vi "arreglos.vi"(0 "Orden":T2(array[ring])=[enum."espejos", enum."voltaje", enum."polarizador", enum."potenciometro ", enum."CCD"], 1 "DISP 1":i32, 2 "Cluster DISP 1":T1, 3 "DISP 2":i32, 4 "DISP 3":i32, 5 "DISPLONG 1":i32, 6 "Cluster DISP 2":T1, 7 "DISPLONG 2":i32, 8 "DISPLONG 3":i32, 9 "nombre":string, 10 "CORRIENTE":dbl[](array[numeric]), 11 "MULTIMETRO 2":dbl[](array[numeric]), 12 "VOLTAJE":dbl[](array[numeric]), 13 "X":dbl[](array[numeric]), 14 "ANGULO":dbl[](array[numeric]), 15 "Y":dbl[](array[numeric]), 16 "laser":dbl[](array[numeric]), 17 "POTENCIOMETRO":dbl[](array[numeric]), 18 "LOCKIN":dbl[](array[numeric]), 19 "CCD":dbl[][](array[numeric]), 20 "MULTIMETRO":bool, 24 "Cluster DISP 4":T1, 27 "Cluster DISP 3":T1) -> (21 "disp 2":T1, 23 "disp 1":T1, 25 "disp 3":T1, 26 "disp 4":T1)   [LabVIEW 2016]
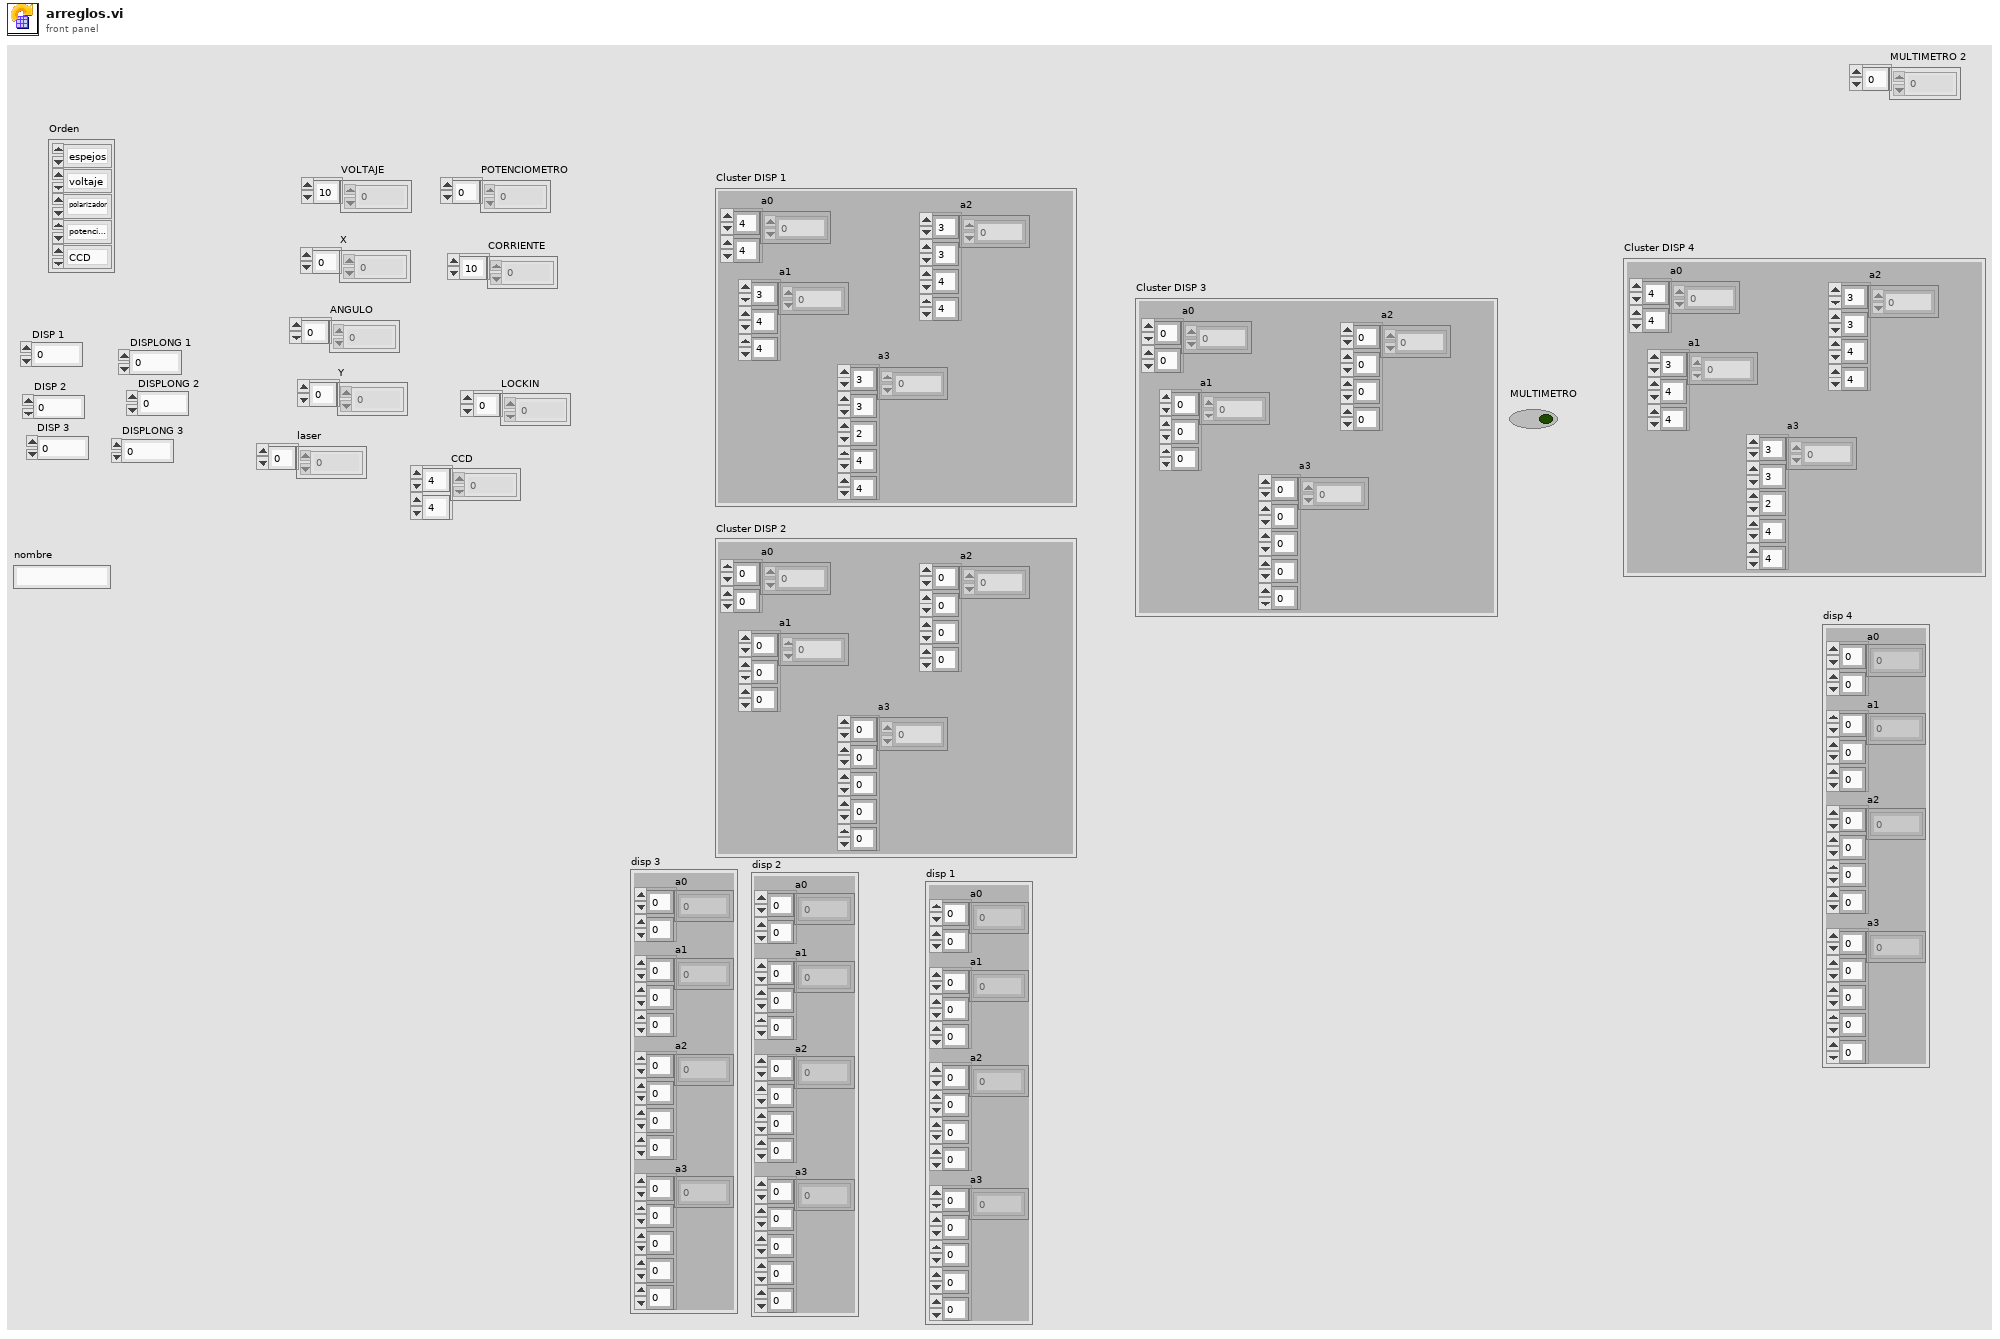
[diagram p1: front panel]
types:
  T1 = cluster{"a0":dbl[][], "a1":dbl[][][], "a2":dbl[][][][], "a3":dbl[][][][][]}
  T2 = enum16{"espejos", "polarizador", "voltaje", "potenciometro ", "CCD", "lockin", "laser", "ninguno"}[]
  T3 = enum16{"espejos", "polarizador", "voltaje", "potenciometro ", "CCD", "lockin", "laser", "ninguno"}
  T4 = enum16{"espejos", "polarizador", "voltaje", "potenciometro ", "CCD", "lockin", "laser", "multimetro", "ninguno"}
  T5 = cluster{"a0":dbl[][], "a1":dbl[][][], "a2":dbl[][][][], "a3":dbl[][][][][]}[]
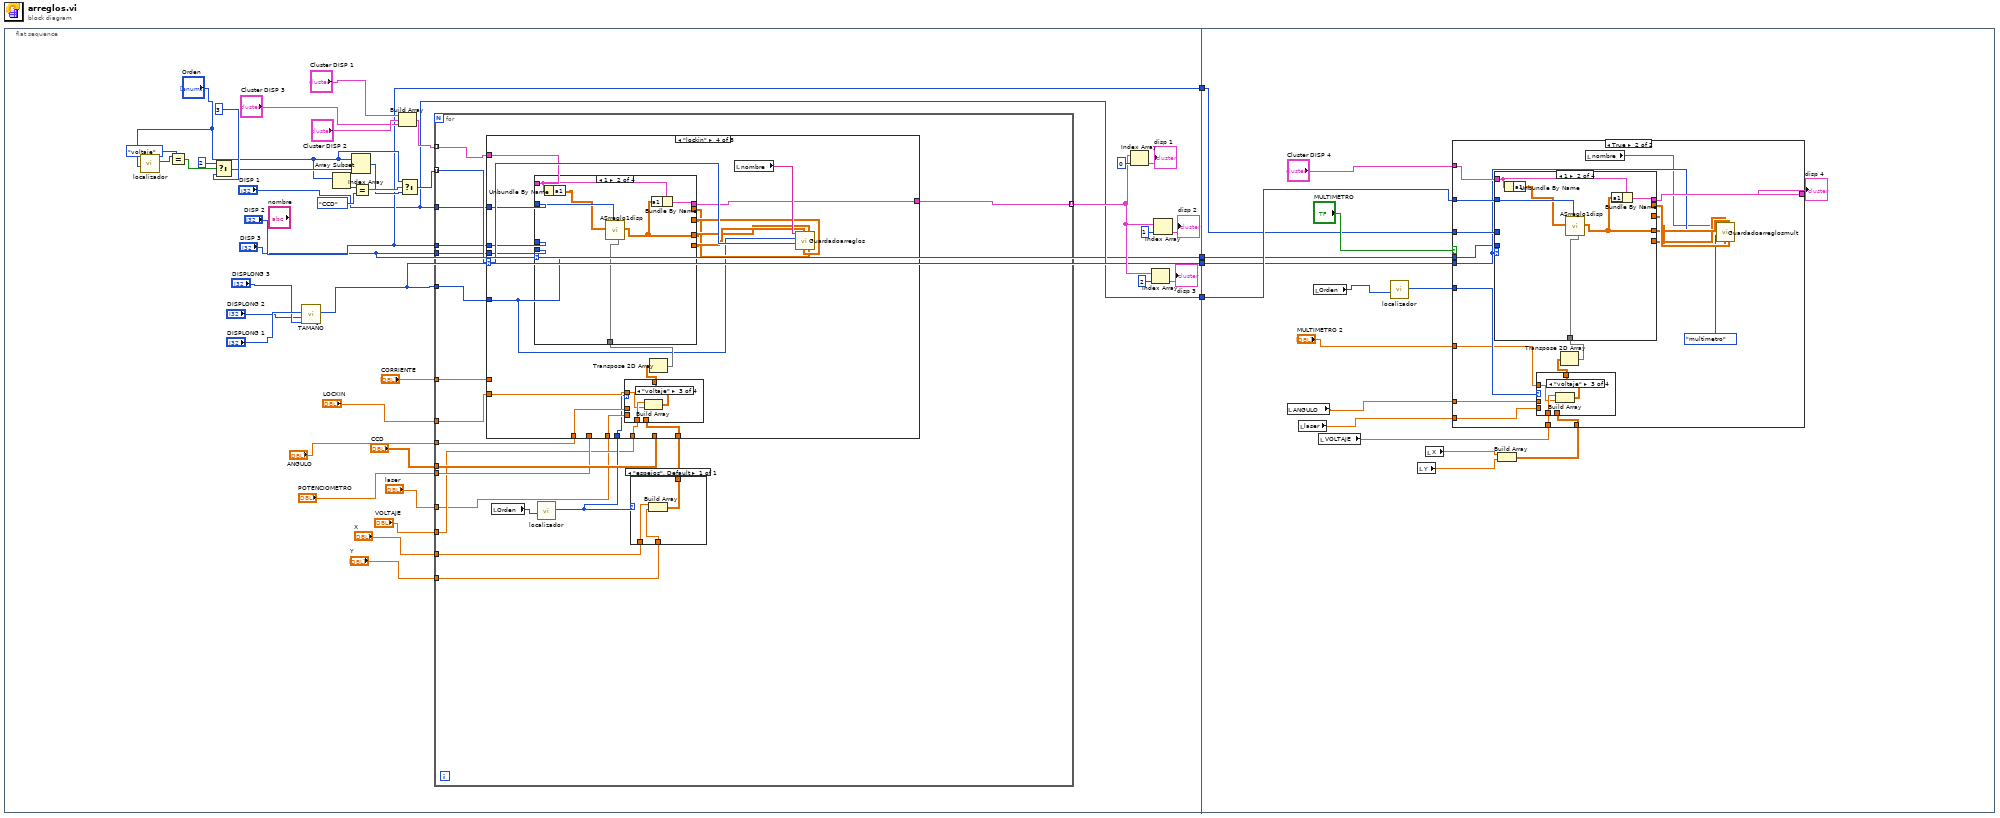
[diagram p0: block diagram]
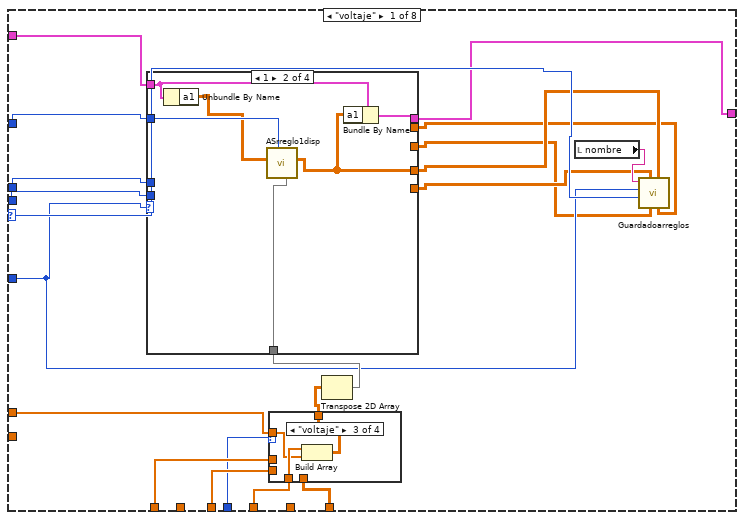
[diagram p2: hidden frame]
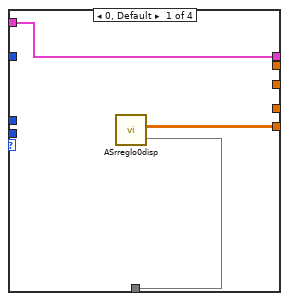
[diagram p3: hidden frame]
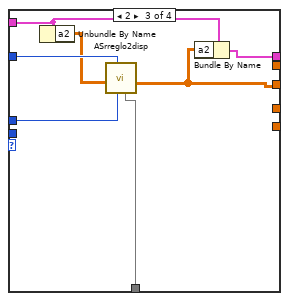
[diagram p4: hidden frame]
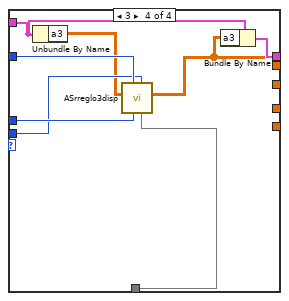
[diagram p5: hidden frame]
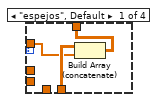
[diagram p6: hidden frame]
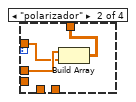
[diagram p7: hidden frame]
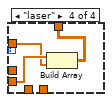
[diagram p8: hidden frame]
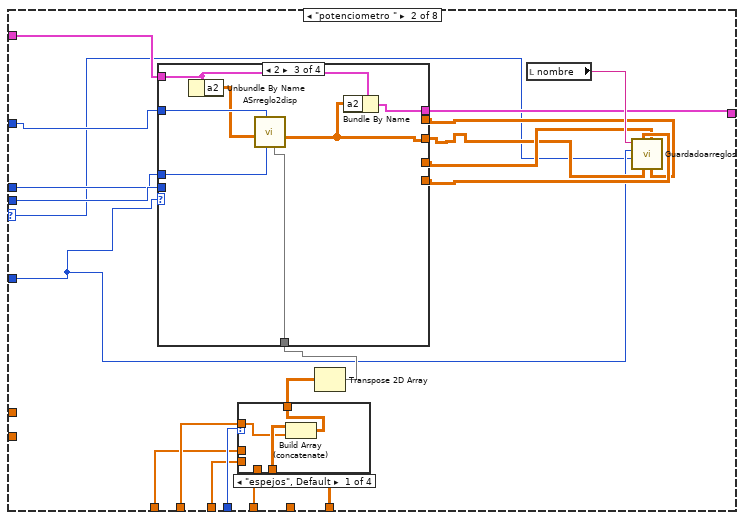
[diagram p9: hidden frame]
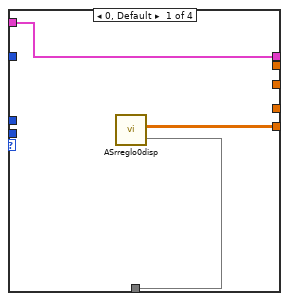
[diagram p10: hidden frame]
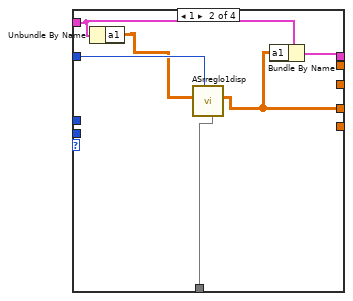
[diagram p11: hidden frame]
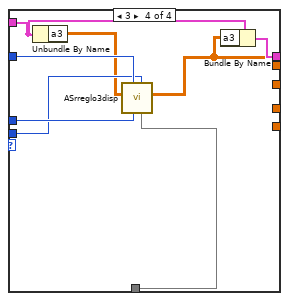
[diagram p12: hidden frame]
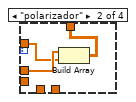
[diagram p13: hidden frame]
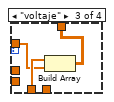
[diagram p14: hidden frame]
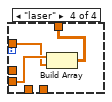
[diagram p15: hidden frame]
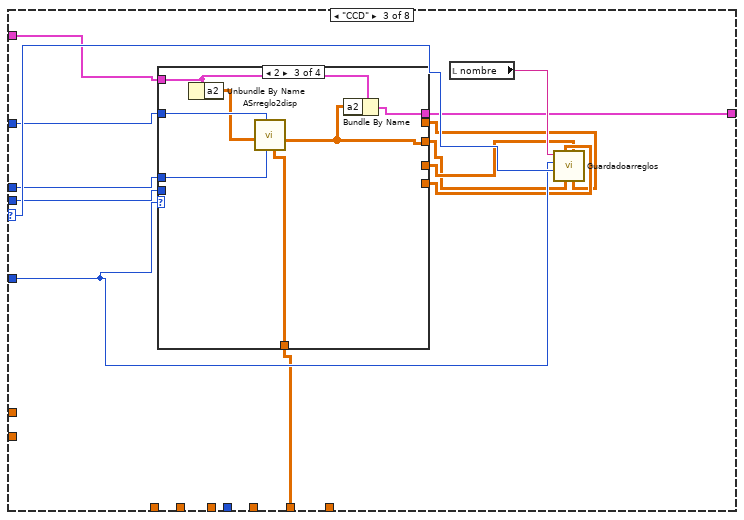
[diagram p16: hidden frame]
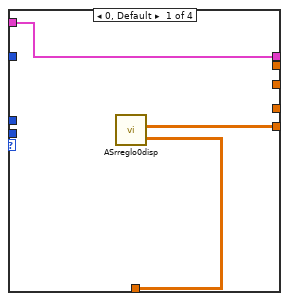
[diagram p17: hidden frame]
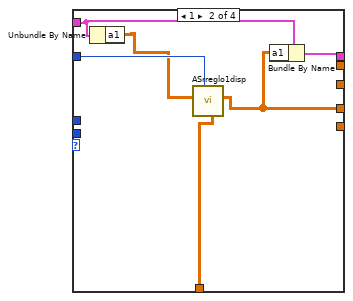
[diagram p18: hidden frame]
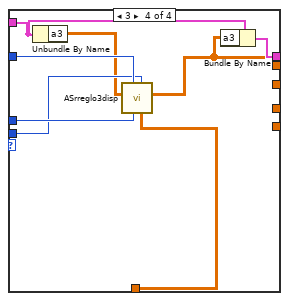
[diagram p19: hidden frame]
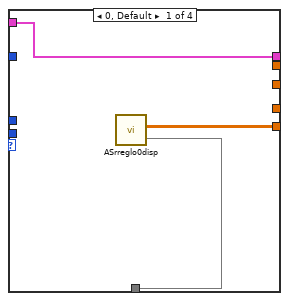
[diagram p20: hidden frame]
diagram:
  n1 = flat-sequence {
    tunnel: ["DISP 1"] -> w4
    tunnel: ["DISP 2"] -> w3
    tunnel: [w7] -> w2
    tunnel: ["DISP 3"] -> w1
    tunnel: w4 -> [w278]
    tunnel: w3 -> [w277]
    tunnel: w2 -> [w276]
    tunnel: w1 -> [w275]
    frame #0 {
      n2 = call "localizador.vi"("Orden"="Orden") -> ("Enum"=w24:T3)  [unwired: 9 in, 1 out]
      n3 = Equal?(x=w24, y=T3."voltaje") -> (x = y?=w22:bool)
      n4 = Select(t=2, s=w22, f=3 ("index")) -> (s? t:f=w20:i32)
      n5 = call "TAMAÑO.vi"("DISPLONG 3"="DISPLONG 3", "DISPLONG 2"="DISPLONG 2", "DISPLONG 1"="DISPLONG 1") -> ("result"=w7:i32)  [unwired: 8 in]
      n6 = Index Array(array="Orden") -> (element=w14:T3)  [unwired: 1 in]
      n7 = Array Subset(array="Orden", index=w20) -> (w10:T2)  [unwired: 1 in]
      n8 = Equal?(x=w14, y=T3."CCD") -> (x = y?=w12:bool)
      n9 = Build Array("Cluster DISP 1", "Cluster DISP 2", "Cluster DISP 3") -> (w29:T5)
      n10 = Select(t="Orden", s=w12, f=w10) -> (s? t:f=w9:T2)
      n11 = for {
        tunnel: w9 -> [w61] mode=indexing
        tunnel: w7 -> [w62]
        tunnel: "CCD" -> [w60]
        tunnel: "DISP 1" -> [w59]
        tunnel: "DISP 2" -> [w58]
        tunnel: "DISP 3" -> [w57]
        tunnel: "POTENCIOMETRO" -> [w56]
        tunnel: "Y" -> [w54]
        tunnel: "X" -> [w53]
        tunnel: "VOLTAJE" -> [w50]
        tunnel: "ANGULO" -> [w49]
        tunnel: "laser" -> [w48]
        tunnel: "LOCKIN" -> [w47]
        tunnel: "CORRIENTE" -> [w46]
        tunnel: w29 -> [w45] mode=indexing
        tunnel: [w44] -> w17 mode=indexing
        n12 = local read "Orden"() -> (w55:T2)
        n13 = call "localizador.vi"("Orden"=w55) -> ("Enum"=w51:T3)  [unwired: 9 in, 1 out]
        n14 = case shown="\"espejos\", Default" w51 {
          tunnel: w54 -> [w64]
          tunnel: w53 -> [w65]
          tunnel: [w63] -> w52
          frame "espejos", Default {
            n15 = Build Array(w65, w64) -> (w63:dbl[][])
          }
        }
        n16 = case shown="\"lockin\"" w61 {
          selector: w61 -> [w77 w122 w189 w226 _ _ _ _]
          tunnel: w62 -> [w75 w126 w185 w215 _ _ _ _]
          tunnel: w60 -> [_ _ w184 _ _ _ _ _]
          tunnel: w59 -> [w72 w123 w188 w223 _ _ _ _]
          tunnel: w58 -> [w73 w124 w187 w225 _ _ _ _]
          tunnel: w57 -> [w74 w125 w186 w224 _ _ _ _]
          tunnel: w56 -> [_ w141 _ _ _ _ _ _]
          tunnel: w52 -> [w80 w140 _ w231 _ _ _ _]
          tunnel: w51 -> [w79 w139 _ w228 _ _ _ _]
          tunnel: w50 -> [w82 w138 _ w229 _ _ _ _]
          tunnel: w49 -> [w84 w136 _ w234 _ _ _ _]
          tunnel: w48 -> [w81 w135 _ w230 _ _ _ _]
          tunnel: w47 -> [_ _ _ w233 _ _ _ _]
          tunnel: w46 -> [w83 _ _ _ _ _ _ _]
          tunnel: w45 -> [w71 w129 w179 w222 w271 w272 w273 w274]
          tunnel: [w70 w128 w178 w221 w271 w272 w273 w274] -> w44
          frame "voltaje" {
            n17 = case shown="\"voltaje\"" w79 {
              tunnel: [w110 w113 w116 w119] -> w85
              tunnel: w83 -> [w111 w114 w117 w120]
              tunnel: w80 -> [w112 _ _ _]
              tunnel: w82 -> [_ _ w118 _]
              tunnel: w84 -> [_ w115 _ _]
              tunnel: w81 -> [_ _ _ w121]
              frame "espejos", Default {
                n18 = Build Array (concatenate)(w112, w111) -> (w110:dbl[][])
              }
              frame "polarizador" {
                n19 = Build Array(w115, w114) -> (w113:dbl[][])
              }
              frame "voltaje" {
                n20 = Build Array(w118, w117) -> (w116:dbl[][])
              }
              frame "laser" {
                n21 = Build Array(w121, w120) -> (w119:dbl[][])
              }
            }
            n22 = Transpose 2D Array(2D array=w85) -> (transposed array=w76:dbl[][])
            n23 = case shown="1" w75 {
              tunnel: [w88 _ _ _] -> w69
              tunnel: w76 -> [w87 w93 w101 w109]
              tunnel: [_ w89 _ _] -> w68
              tunnel: [_ _ w97 _] -> w67
              tunnel: [_ _ _ w102] -> w66
              tunnel: w72 -> [_ w94 w100 w107]
              tunnel: w73 -> [_ _ w95 w108]
              tunnel: w74 -> [_ _ _ w106]
              tunnel: w71 -> [w86 w90 w98 w103]
              tunnel: [w86 w91 w96 w104] -> w70
              frame 0, Default {
                n24 = call "ASrreglo0disp.vi"("datos"=w87) -> ("output array"=w88:dbl[][])  [unwired: 10 in]
              }
              frame 1 {
                n25 = Unbundle By Name(w90) -> ("a1"=w92:dbl[][][])
                n26 = call "ASrreglo1disp.vi"("datos"=w93, "disp. 1"=w94, "ARREGLO ENTRADA"=w92) -> ("output array"=w89:dbl[][][])  [unwired: 8 in]
                n27 = Bundle By Name(cluster=w90, "a1"=w89) -> (w91:T1)
              }
              frame 2 {
                n28 = Unbundle By Name(w98) -> ("a2"=w99:dbl[][][][])
                n29 = call "ASrreglo2disp.vi"("datos"=w101, "disp. 2"=w95, "disp. 1"=w100, "arreglo entrada"=w99) -> ("output array"=w97:dbl[][][][])  [unwired: 7 in]
                n30 = Bundle By Name(cluster=w98, "a2"=w97) -> (w96:T1)
              }
              frame 3 {
                n31 = Unbundle By Name(w103) -> ("a3"=w105:dbl[][][][][])
                n32 = call "ASrreglo3disp.vi"("datos"=w109, "disp. 3"=w106, "disp. 2"=w108, "disp. 1"=w107, "output array 2"=w105) -> ("output array"=w102:dbl[][][][][])  [unwired: 6 in]
                n33 = Bundle By Name(cluster=w103, "a3"=w102) -> (w104:T1)
              }
            }
            n34 = local read "nombre"() -> (w78:string)
            n35 = call "Guardadoarreglos.vi"("disp 3"=w66, "disp 1"=w68, "disp 2"=w67, "disp 0"=w69, "Enum"=w77, "indice"=w75, "nombre"=w78) -> ()  [unwired: 5 in]
          }
          frame "potenciometro " {
            n36 = case shown="\"espejos\", Default" w139 {
              tunnel: [w166 w169 w172 w175] -> w137
              tunnel: w141 -> [w167 w170 w173 w176]
              tunnel: w140 -> [w168 _ _ _]
              tunnel: w138 -> [_ _ w174 _]
              tunnel: w136 -> [_ w171 _ _]
              tunnel: w135 -> [_ _ _ w177]
              frame "espejos", Default {
                n37 = Build Array (concatenate)(w168, w167) -> (w166:dbl[][])
              }
              frame "polarizador" {
                n38 = Build Array(w171, w170) -> (w169:dbl[][])
              }
              frame "voltaje" {
                n39 = Build Array(w174, w173) -> (w172:dbl[][])
              }
              frame "laser" {
                n40 = Build Array(w177, w176) -> (w175:dbl[][])
              }
            }
            n41 = Transpose 2D Array(2D array=w137) -> (transposed array=w127:dbl[][])
            n42 = case shown="2" w126 {
              tunnel: [w144 _ _ _] -> w133
              tunnel: w127 -> [w143 w149 w157 w165]
              tunnel: [_ w145 _ _] -> w132
              tunnel: [_ _ w153 _] -> w131
              tunnel: [_ _ _ w158] -> w130
              tunnel: w123 -> [_ w150 w156 w163]
              tunnel: w124 -> [_ _ w151 w164]
              tunnel: w125 -> [_ _ _ w162]
              tunnel: w129 -> [w142 w146 w154 w159]
              tunnel: [w142 w147 w152 w160] -> w128
              frame 0, Default {
                n43 = call "ASrreglo0disp.vi"("datos"=w143) -> ("output array"=w144:dbl[][])  [unwired: 10 in]
              }
              frame 1 {
                n44 = Unbundle By Name(w146) -> ("a1"=w148:dbl[][][])
                n45 = call "ASrreglo1disp.vi"("datos"=w149, "disp. 1"=w150, "ARREGLO ENTRADA"=w148) -> ("output array"=w145:dbl[][][])  [unwired: 8 in]
                n46 = Bundle By Name(cluster=w146, "a1"=w145) -> (w147:T1)
              }
              frame 2 {
                n47 = Unbundle By Name(w154) -> ("a2"=w155:dbl[][][][])
                n48 = call "ASrreglo2disp.vi"("datos"=w157, "disp. 2"=w151, "disp. 1"=w156, "arreglo entrada"=w155) -> ("output array"=w153:dbl[][][][])  [unwired: 7 in]
                n49 = Bundle By Name(cluster=w154, "a2"=w153) -> (w152:T1)
              }
              frame 3 {
                n50 = Unbundle By Name(w159) -> ("a3"=w161:dbl[][][][][])
                n51 = call "ASrreglo3disp.vi"("datos"=w165, "disp. 3"=w162, "disp. 2"=w164, "disp. 1"=w163, "output array 2"=w161) -> ("output array"=w158:dbl[][][][][])  [unwired: 6 in]
                n52 = Bundle By Name(cluster=w159, "a3"=w158) -> (w160:T1)
              }
            }
            n53 = local read "nombre"() -> (w134:string)
            n54 = call "Guardadoarreglos.vi"("disp 3"=w130, "disp 1"=w132, "disp 2"=w131, "disp 0"=w133, "Enum"=w122, "indice"=w126, "nombre"=w134) -> ()  [unwired: 5 in]
          }
          frame "CCD" {
            n55 = case shown="2" w185 {
              tunnel: [w193 _ _ _] -> w183
              tunnel: w184 -> [w192 w198 w206 w214]
              tunnel: [_ w194 _ _] -> w182
              tunnel: [_ _ w202 _] -> w181
              tunnel: [_ _ _ w207] -> w180
              tunnel: w188 -> [_ w199 w205 w212]
              tunnel: w187 -> [_ _ w200 w213]
              tunnel: w186 -> [_ _ _ w211]
              tunnel: w179 -> [w191 w195 w203 w208]
              tunnel: [w191 w196 w201 w209] -> w178
              frame 0, Default {
                n56 = call "ASrreglo0disp.vi"("datos"=w192) -> ("output array"=w193:dbl[][])  [unwired: 10 in]
              }
              frame 1 {
                n57 = Unbundle By Name(w195) -> ("a1"=w197:dbl[][][])
                n58 = call "ASrreglo1disp.vi"("datos"=w198, "disp. 1"=w199, "ARREGLO ENTRADA"=w197) -> ("output array"=w194:dbl[][][])  [unwired: 8 in]
                n59 = Bundle By Name(cluster=w195, "a1"=w194) -> (w196:T1)
              }
              frame 2 {
                n60 = Unbundle By Name(w203) -> ("a2"=w204:dbl[][][][])
                n61 = call "ASrreglo2disp.vi"("datos"=w206, "disp. 2"=w200, "disp. 1"=w205, "arreglo entrada"=w204) -> ("output array"=w202:dbl[][][][])  [unwired: 7 in]
                n62 = Bundle By Name(cluster=w203, "a2"=w202) -> (w201:T1)
              }
              frame 3 {
                n63 = Unbundle By Name(w208) -> ("a3"=w210:dbl[][][][][])
                n64 = call "ASrreglo3disp.vi"("datos"=w214, "disp. 3"=w211, "disp. 2"=w213, "disp. 1"=w212, "output array 2"=w210) -> ("output array"=w207:dbl[][][][][])  [unwired: 6 in]
                n65 = Bundle By Name(cluster=w208, "a3"=w207) -> (w209:T1)
              }
            }
            n66 = local read "nombre"() -> (w190:string)
            n67 = call "Guardadoarreglos.vi"("disp 3"=w180, "disp 1"=w182, "disp 2"=w181, "disp 0"=w183, "Enum"=w189, "indice"=w185, "nombre"=w190) -> ()  [unwired: 5 in]
          }
          frame "lockin" {
            n68 = case shown="\"voltaje\"" w228 {
              tunnel: [w259 w262 w265 w268] -> w232
              tunnel: w233 -> [w260 w263 w266 w269]
              tunnel: w231 -> [w261 _ _ _]
              tunnel: w229 -> [_ _ w267 _]
              tunnel: w234 -> [_ w264 _ _]
              tunnel: w230 -> [_ _ _ w270]
              frame "espejos", Default {
                n69 = Build Array (concatenate)(w261, w260) -> (w259:dbl[][])
              }
              frame "polarizador" {
                n70 = Build Array(w264, w263) -> (w262:dbl[][])
              }
              frame "voltaje" {
                n71 = Build Array(w267, w266) -> (w265:dbl[][])
              }
              frame "laser" {
                n72 = Build Array(w270, w269) -> (w268:dbl[][])
              }
            }
            n73 = Transpose 2D Array(2D array=w232) -> (transposed array=w220:dbl[][])
            n74 = case shown="1" w215 {
              tunnel: [w237 _ _ _] -> w219
              tunnel: w220 -> [w236 w242 w250 w258]
              tunnel: [_ w238 _ _] -> w218
              tunnel: [_ _ w246 _] -> w217
              tunnel: [_ _ _ w251] -> w216
              tunnel: w223 -> [_ w243 w249 w256]
              tunnel: w225 -> [_ _ w244 w257]
              tunnel: w224 -> [_ _ _ w255]
              tunnel: w222 -> [w235 w239 w247 w252]
              tunnel: [w235 w240 w245 w253] -> w221
              frame 0, Default {
                n75 = call "ASrreglo0disp.vi"("datos"=w236) -> ("output array"=w237:dbl[][])  [unwired: 10 in]
              }
              frame 1 {
                n76 = Unbundle By Name(w239) -> ("a1"=w241:dbl[][][])
                n77 = call "ASrreglo1disp.vi"("datos"=w242, "disp. 1"=w243, "ARREGLO ENTRADA"=w241) -> ("output array"=w238:dbl[][][])  [unwired: 8 in]
                n78 = Bundle By Name(cluster=w239, "a1"=w238) -> (w240:T1)
              }
              frame 2 {
                n79 = Unbundle By Name(w247) -> ("a2"=w248:dbl[][][][])
                n80 = call "ASrreglo2disp.vi"("datos"=w250, "disp. 2"=w244, "disp. 1"=w249, "arreglo entrada"=w248) -> ("output array"=w246:dbl[][][][])  [unwired: 7 in]
                n81 = Bundle By Name(cluster=w247, "a2"=w246) -> (w245:T1)
              }
              frame 3 {
                n82 = Unbundle By Name(w252) -> ("a3"=w254:dbl[][][][][])
                n83 = call "ASrreglo3disp.vi"("datos"=w258, "disp. 3"=w255, "disp. 2"=w257, "disp. 1"=w256, "output array 2"=w254) -> ("output array"=w251:dbl[][][][][])  [unwired: 6 in]
                n84 = Bundle By Name(cluster=w252, "a3"=w251) -> (w253:T1)
              }
            }
            n85 = local read "nombre"() -> (w227:string)
            n86 = call "Guardadoarreglos.vi"("disp 3"=w216, "disp 1"=w218, "disp 2"=w217, "disp 0"=w219, "Enum"=w226, "indice"=w215, "nombre"=w227) -> ()  [unwired: 5 in]
          }
          frame "laser" {
          }
          frame "ninguno", Default {
          }
          frame "polarizador" {
          }
          frame "espejos" {
          }
        }
      }
      n87 = Index Array(array=w17, index=0) -> (element=→"disp 1":T1)
      n88 = Index Array(array=w17, index=2) -> (element=→"disp 3":T1)
      n89 = Index Array(array=w17, index=1) -> (element=→"disp 2":T1)
    }
    frame #1 {
      n90 = local read "ANGULO"() -> (w279:dbl[])
      n91 = local read "laser"() -> (w280:dbl[])
      n92 = local read "Orden"() -> (w284:T2)
      n93 = local read "VOLTAJE"() -> (w281:dbl[])
      n94 = call "localizador.vi"("Orden"=w284) -> ("Enum"=w288:T3)  [unwired: 9 in, 1 out]
      n95 = local read "Y"() -> (w282:dbl[])
      n96 = local read "X"() -> (w283:dbl[])
      n97 = Build Array(w283, w282) -> (w287:dbl[][])
      n98 = case shown="True" "MULTIMETRO" {
        tunnel: "Cluster DISP 4" -> [w291 w311]
        tunnel: [w291 w310] -> w286
        tunnel: w278 -> [_ w309]
        tunnel: w277 -> [_ w308]
        tunnel: w276 -> [_ w294]
        tunnel: "MULTIMETRO 2" -> [_ w304]
        tunnel: w288 -> [_ w305]
        tunnel: w279 -> [_ w303]
        tunnel: w280 -> [_ w302]
        tunnel: w281 -> [_ w301]
        tunnel: w287 -> [_ w300]
        tunnel: w275 -> [_ w292]
        frame False {
        }
        frame True {
          n99 = case shown="\"voltaje\"" w305 {
            tunnel: [w312 w315 w318 w321] -> w307
            tunnel: w304 -> [w313 w316 w319 w322]
            tunnel: w300 -> [w314 _ _ _]
            tunnel: w301 -> [_ _ w320 _]
            tunnel: w303 -> [_ w317 _ _]
            tunnel: w302 -> [_ _ _ w323]
            frame "espejos", Default {
              n100 = Build Array (concatenate)(w314, w313) -> (w312:dbl[][])
            }
            frame "polarizador" {
              n101 = Build Array(w317, w316) -> (w315:dbl[][])
            }
            frame "voltaje" {
              n102 = Build Array(w320, w319) -> (w318:dbl[][])
            }
            frame "laser" {
              n103 = Build Array(w323, w322) -> (w321:dbl[][])
            }
          }
          n104 = Transpose 2D Array(2D array=w307) -> (transposed array=w306:dbl[][])
          n105 = case shown="1" w294 {
            tunnel: [w326 _ _ _] -> w296
            tunnel: w306 -> [w325 w331 w338 w346]
            tunnel: [_ w327 _ _] -> w297
            tunnel: [_ _ w334 _] -> w298
            tunnel: [_ _ _ w340] -> w299
            tunnel: w309 -> [_ w332 w337 w345]
            tunnel: w292 -> [_ _ _ w344]
            tunnel: w311 -> [w324 w328 w335 w341]
            tunnel: [w324 w329 w333 w342] -> w310
            tunnel: w308 -> [_ _ _ w339]
            frame 0, Default {
              n106 = call "ASrreglo0disp.vi"("datos"=w325) -> ("output array"=w326:dbl[][])  [unwired: 10 in]
            }
            frame 1 {
              n107 = Unbundle By Name(w328) -> ("a1"=w330:dbl[][][])
              n108 = call "ASrreglo1disp.vi"("datos"=w331, "disp. 1"=w332, "ARREGLO ENTRADA"=w330) -> ("output array"=w327:dbl[][][])  [unwired: 8 in]
              n109 = Bundle By Name(cluster=w328, "a1"=w327) -> (w329:T1)
            }
            frame 2 {
              n110 = Unbundle By Name(w335) -> ("a2"=w336:dbl[][][][])
              n111 = call "ASrreglo2disp.vi"("datos"=w338, "disp. 1"=w337, "arreglo entrada"=w336) -> ("output array"=w334:dbl[][][][])  [unwired: 8 in]
              n112 = Bundle By Name(cluster=w335, "a2"=w334) -> (w333:T1)
            }
            frame 3 {
              n113 = Unbundle By Name(w341) -> ("a3"=w343:dbl[][][][][])
              n114 = call "ASrreglo3disp.vi"("datos"=w346, "disp. 3"=w344, "disp. 2"=w339, "disp. 1"=w345, "output array 2"=w343) -> ("output array"=w340:dbl[][][][][])  [unwired: 6 in]
              n115 = Bundle By Name(cluster=w341, "a3"=w340) -> (w342:T1)
            }
          }
          n116 = local read "nombre"() -> (w293:string)
          n117 = call "Guardadoarreglosmult.vi"("disp 3"=w299, "disp 1"=w297, "disp 2"=w298, "disp 0"=w296, "Enum"=T4."multimetro", "indice"=w294, "nombre"=w293) -> ()  [unwired: 5 in]
        }
      }
      "disp 4" <- w286
    }
  }
